vi "ETH6_E2A_Ref-V.vi"(10 "Ref voltage":dbl, 11 "Write/Read":enum16{"Write", "Read"}(ring)=enum."Read") -> (2 "Ref voltage Out":dbl)   [LabVIEW 2022 SP3]
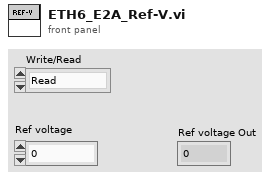
[diagram p1: front panel]
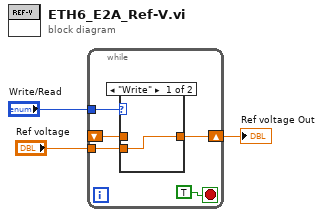
[diagram p0: block diagram]
diagram:
  n1 = while {
    shift-right: [w7] -> w1
    shift-left: _ -> [w5]
    tunnel: "Write/Read" -> [w8]
    tunnel: "Ref voltage" -> [w6]
    stop <- TRUE stop-if-true
    n2 = case shown="\"Write\"" w8 {
      tunnel: w6 -> [w9 _]
      tunnel: [w9 w10] -> w7
      tunnel: w5 -> [_ w10]
      frame "Write" {
      }
      frame "Read", Default {
      }
    }
  }
  "Ref voltage Out" <- w1
